vi "HEWH EMV Startup Control.vi"(5 "Disable EMV GEA Flow":bool, 6 "EMV Position":i16=-200, 7 "State":T1, 8 "error in (no error)":errorcluster, 9 "Manual Mode Time (sec)":dbl=10.0 format="%#_13g", 10 "Elapsed Time (sec)":dbl, 11 ".NET Refnum in":refnum<k24>) -> (0 "error out":errorcluster)   [LabVIEW 2019]
uses:
  Type Definitions/HEWH Purge Draw.ctl
  C:/TechnologyLab/NI-2010/Drivers/GEA3 Toolkit/GEA3 DLL Source/GeaCommunication.dll
  Drivers/GEA3 Toolkit/GEA3 DLL Source/GeaCommunication.dll
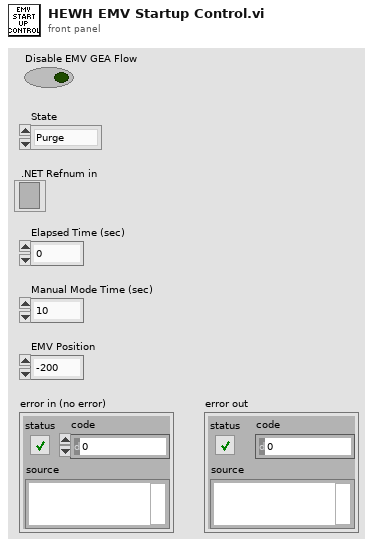
[diagram p1: front panel]
types:
  T1 = typedef "HEWH Purge Draw.ctl" = enum16{"Purge", "Draw"}
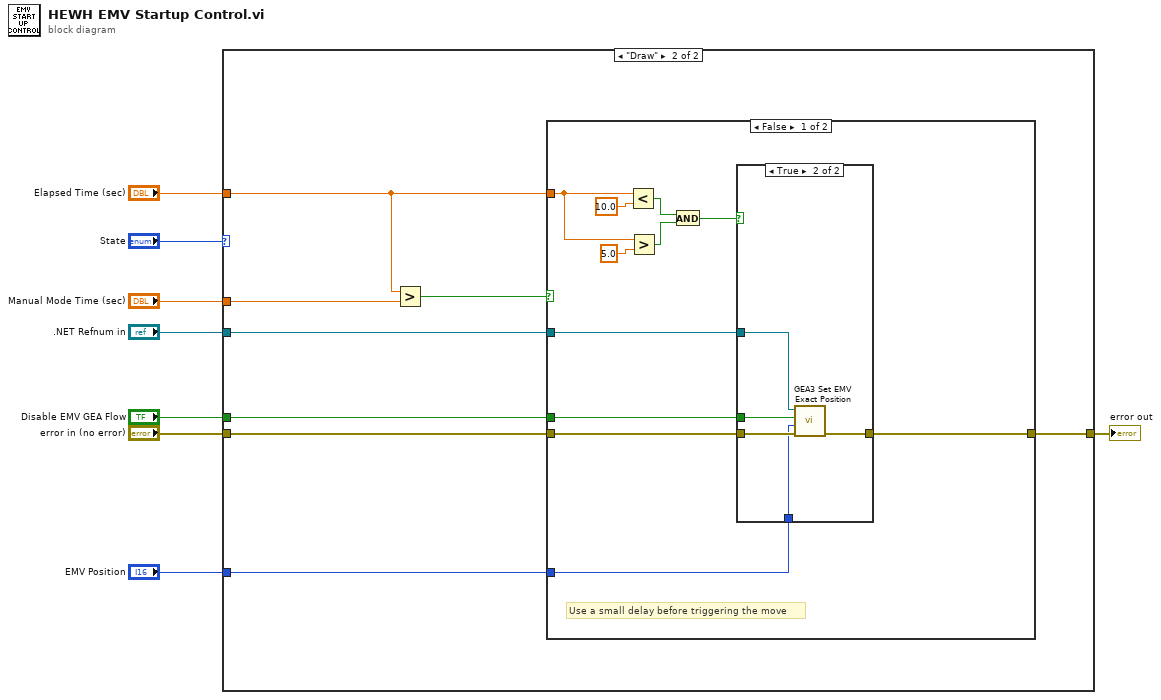
[diagram p0: block diagram]
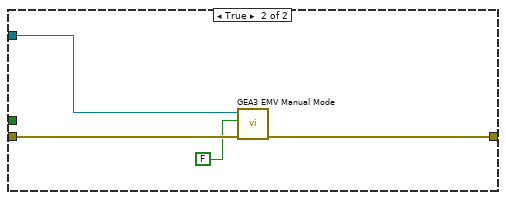
[diagram p4: hidden frame]
diagram:
  n1 = case shown="\"Draw\"" "State" {
    tunnel: "error in (no error)" -> [w9 w17]
    tunnel: [w9 w16] -> w4
    tunnel: ".NET Refnum in" -> [_ w15]
    tunnel: "Elapsed Time (sec)" -> [_ w10]
    tunnel: "Disable EMV GEA Flow" -> [_ w13]
    tunnel: "EMV Position" -> [_ w12]
    tunnel: "Manual Mode Time (sec)" -> [_ w11]
    frame "Purge", Default {
    }
    frame "Draw" {
      n2 = Greater?(x=w10, y=w11) -> (0:w14:bool)
      n3 = case shown="False" w14 {
        tunnel: w17 -> [w28 w37]
        tunnel: [w27 w38] -> w16
        tunnel: w15 -> [w26 w36]
        tunnel: w13 -> [w25 _]
        tunnel: w12 -> [w24 _]
        tunnel: w10 -> [w22 _]
        frame False {
          # "Use a small delay before triggering the move"
          n4 = Less?(x=w22, y=10.0) -> (x < y?=w20:bool)
          n5 = Greater?(x=w22, y=5.0) -> (0:w19:bool)
          n6 = And(x=w20, y=w19) -> (x .and. y?=w18:bool)
          n7 = case shown="True" w18 {
            tunnel: w28 -> [w29 w34]
            tunnel: [w29 w33] -> w27
            tunnel: w26 -> [_ w32]
            tunnel: w25 -> [_ w31]
            tunnel: w24 -> [_ w30]
            frame False {
            }
            frame True {
              n8 = call "GEA3 Set EMV Exact Position.vi"("error in (no error)"=w34, "EMV Position"=w30, "Disable EMV GEA Flow"=w31, ".NET Refnum in"=w32) -> ("error out"=w33:errorcluster)  [unwired: 4 in, 3 out]
            }
          }
        }
        frame True {
          n9 = call "GEA3 EMV Manual Mode.vi"("error in (no error)"=w37, "Manual Mode?"=FALSE, ".NET Refnum in"=w36) -> ("error out"=w38:errorcluster)  [unwired: 7 in, 1 out]
        }
      }
    }
  }
  "error out" <- w4
